vi "SubMeanOfMean.vi"(6 "attn_dB":dbl[](array[numeric]), 7 "means":dbl[][](array[numeric]), 8 "A/D info.# A/D bits":i16, 11 "Scan Data In":dbl[][](array[numeric])) -> (3 "Scan Out":dbl[][](array[numeric]))   [LabVIEW 2022 SP3]
uses:
  <vilib>/Analysis/baseanly.llb/Mean (DBL).vi
  <vilib>/Analysis/NI_AALBase.lvlib
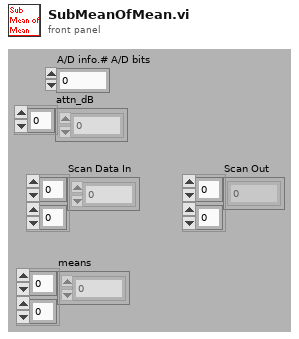
[diagram p1: front panel]
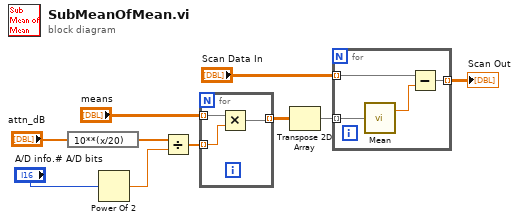
[diagram p0: block diagram]
diagram:
  n1 = expression code="10**(x/20)"("attn_dB") -> (w9:dbl[])
  n2 = Power Of 2(x="A/D info.# A/D bits") -> (2^x=w7:dbl)
  n3 = Divide(x=w9, y=w7) -> (x/y=w5:dbl[])
  n4 = for {
    tunnel: "means" -> [w12] mode=indexing
    tunnel: w5 -> [w13] mode=indexing
    tunnel: [w11] -> w4 mode=indexing
    n5 = Multiply(x=w12, y=w13) -> (x*y=w11:dbl[])
  }
  n6 = Transpose 2D Array(2D array=w4) -> (transposed array=w3:dbl[][])
  n7 = for {
    tunnel: w3 -> [w17] mode=indexing
    tunnel: "Scan Data In" -> [w16] mode=indexing
    tunnel: [w14] -> w2 mode=indexing
    n8 = call-poly <vilib>:"Mean.vi"("X"=w17) -> ("mean"=w15:dbl)  [unwired: 1 out]
    n9 = Subtract(x=w16, y=w15) -> (x-y=w14:dbl[])
  }
  "Scan Out" <- w2
